vi "mqttServer.vi"() -> ()   [LabVIEW 2019]
uses:
  <vilib>/LabVIEW Open Source Project/MQTT Connection/MQTT_Base/Base Class/MQTT_Base.lvclass/MQTT_Base.ctl
  <vilib>/LabVIEW Open Source Project/MQTT Broker/Server class/Server.lvclass/Server.ctl
  <vilib>/LabVIEW Open Source Project/MQTT Control Packets/Control Packets/PUBLISH/PUBLISH.lvclass
  C:/Program Files (x86)/National Instruments/LabVIEW 2019/vi.lib/LabVIEW Open Source Project/MQTT Control Packets/Control Packets/ControlPacket/ControlPacket.lvclass
  <vilib>/LabVIEW Open Source Project/MQTT Control Packets/Control Packets/ControlPacket/ControlPacket.lvclass/ControlPacket.ctl
  <vilib>/LabVIEW Open Source Project/MQTT TCP Connection/MQTT_TCP/Connection/TCPConnection.lvclass
  C:/Program Files (x86)/National Instruments/LabVIEW 2019/vi.lib/LabVIEW Open Source Project/MQTT Connection/MQTT_Connection/Connection/Connection.lvclass
  <vilib>/LabVIEW Open Source Project/MQTT Broker/Server class/Server.lvclass
  C:/Program Files (x86)/National Instruments/LabVIEW 2019/vi.lib/LabVIEW Open Source Project/MQTT Connection/MQTT_Base/Base Class/MQTT_Base.lvclass
  <vilib>/LabVIEW Open Source Project/Epoch Date & Time/epoch.UNIX/Epoch.UNIX.lvclass
  C:/Program Files (x86)/National Instruments/LabVIEW 2019/vi.lib/LabVIEW Open Source Project/Epoch Date & Time/epoch/Epoch.lvclass
  <vilib>/LabVIEW Open Source Project/Epoch Date & Time/Get Epoch Time.vi
  <vilib>/LabVIEW Open Source Project/MQTT Connection/MQTT_Base/Base Class/MQTT_Base.lvclass
  <vilib>/LabVIEW Open Source Project/MQTT Control Packets/Control Packets/ControlPacket/ControlPacket.lvclass
panel:
  in  "Trace Messages":bool
  out "Error Server":errorcluster
  out "NbConnections":u32
  out "Inbound Log":string
  in  "AutoScroll":bool=TRUE
  in  "Clear Log":bool
  # "Native LabVIEW MQTT Broker"
  # "G Open Source Project for LabVIEW\nhttps://github.com/LabVIEW-Open-Source/LV-MQTT-Broker"
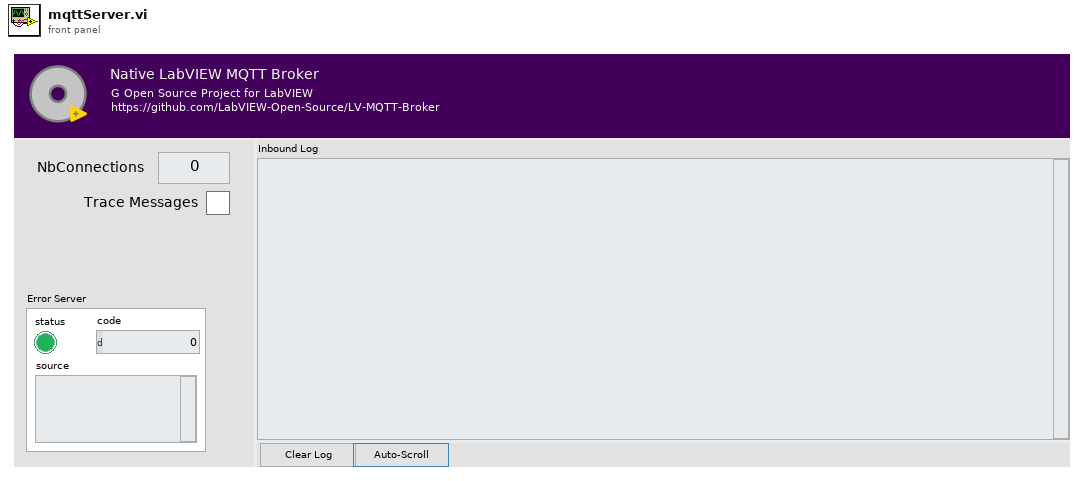
[diagram p1: front panel]
types:
  T1 = typedef "MQTT Base.lvlib/MQTT_Base.lvclass/Public Events -- cluster.ctl" = cluster{"Stop Event":refnum<user-event>, "Error Event":refnum<user-event>, "Inbound Message":refnum<user-event>}
  T2 = typedef "MQTT Server.lvlib/Server.lvclass/Public Events -- cluster.ctl" = cluster{"NbConnections":refnum<user-event>}
  T3 = typedef "MQTT_Control_Packets.lvlib/ControlPacket.lvclass/QualityOfService -- enum.ctl" = enum16{"0 (At Most Once)", "1 (At Least Once)", "2 (Exactly Once)"}
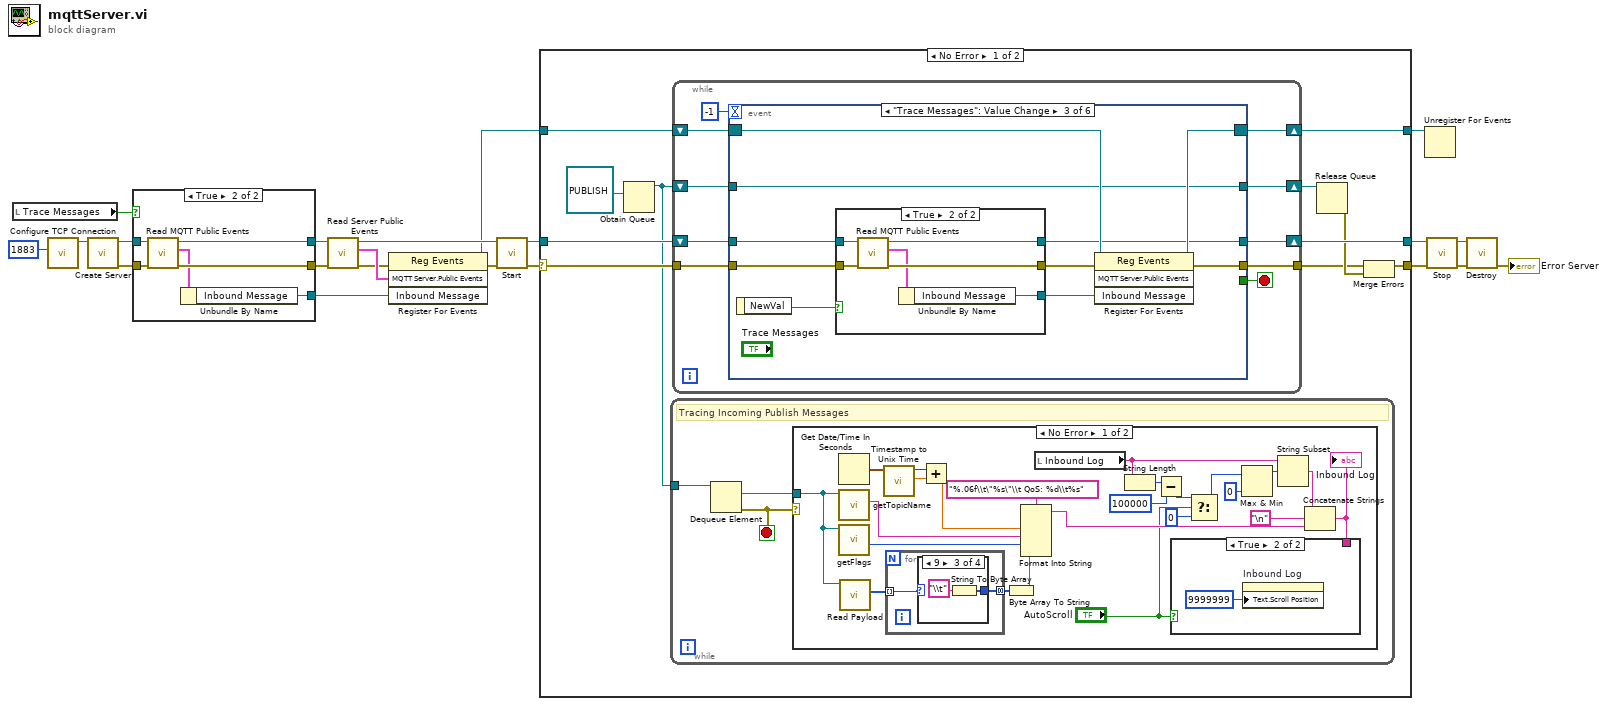
[diagram p0: block diagram]
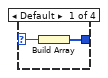
[diagram p4: hidden frame]
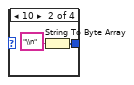
[diagram p5: hidden frame]
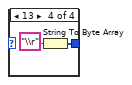
[diagram p6: hidden frame]
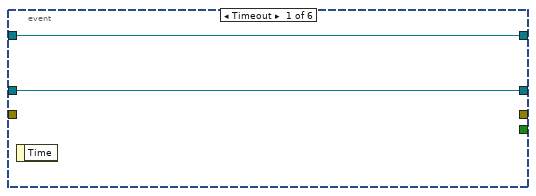
[diagram p8: hidden frame]
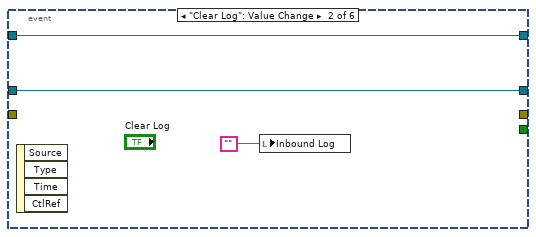
[diagram p9: hidden frame]
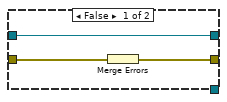
[diagram p10: hidden frame]
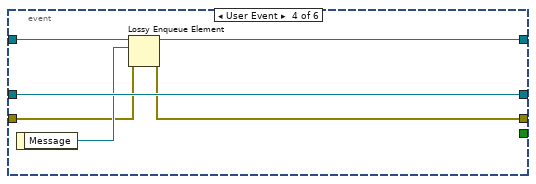
[diagram p11: hidden frame]
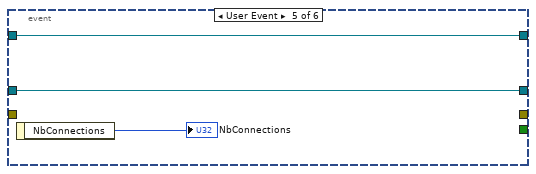
[diagram p12: hidden frame]
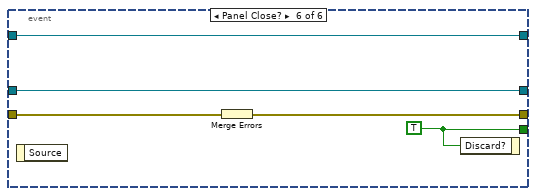
[diagram p13: hidden frame]
diagram:
  n1 = local read "Trace Messages"() -> (w1:bool)
  n2 = call <vilib>:"Configure TCP Connection.vi"("remote port (80)"=u16 1883) -> ("TCPConnection"=w7:refnum<class "TCPConnection.lvclass">)  [unwired: 9 in, 1 out]
  n3 = call <vilib>:"Create Server.vi"("Connection Configuration"=w7) -> ("error out"=w6:errorcluster, "Server"=w4:refnum<class "Server.lvclass">)  [unwired: 9 in]
  n4 = case shown="True" w1 {
    tunnel: w6 -> [w22 w29]
    tunnel: [w22 w28] -> w5
    tunnel: w4 -> [w23 w27]
    tunnel: [w23 w26] -> w3
    tunnel: [_ w24] -> w2
    frame False {
    }
    frame True {
      n5 = call <vilib>:"Read MQTT Public Events.vi"("error in (no error)"=w29, "MQTT_Base in"=w27) -> ("error out"=w28:errorcluster, "MQTT Public Events"=w25:T1, "MQTT_Base out"=w26:refnum<class "Server.lvclass">)  [unwired: 7 in]
      n6 = Unbundle By Name(w25) -> ("Inbound Message"=w24:refnum<user-event>)
    }
  }
  n7 = call <vilib>:"Read Server Public Events.vi"("error in (no error)"=w5, "Server in"=w3) -> ("error out"=w9:errorcluster, "MQTT Server.Public Events"=w10:T2, "Server out"=w13:refnum<class "Server.lvclass">)  [unwired: 7 in]
  n8 = register-events(error in=w9, w10, w2) -> (reference out=w11:refnum<event-registration>, error out=w15:errorcluster)  [unwired: 1 in]
  n9 = call <vilib>:"Start.vi"("error in (no error)"=w15, "MQTT_Base in"=w13) -> ("error out"=w16:errorcluster, "MQTT_Base out"=w14:refnum<class "Server.lvclass">)  [unwired: 7 in, 1 out]
  n10 = case shown="No Error" w16 {
    selector: w16 -> [w36 w127]
    tunnel: w14 -> [w40 w129]
    tunnel: [w39 w129] -> w19
    tunnel: w11 -> [w38 w128]
    tunnel: [w37 w128] -> w12
    tunnel: [w32 w127] -> w21
    frame No Error {
      n11 = Obtain Queue(element data type=refnum<class "PUBLISH.lvclass"> refnum ("Message")) -> (queue out=w31:refnum<queue>)  [unwired: 4 in, 2 out]
      n12 = while {
        tunnel: w31 -> [w43]
        stop <- w42 stop-if-true
        # "Tracing Incoming Publish Messages"
        n13 = Dequeue Element(queue=w43) -> (element=w41:refnum<class "PUBLISH.lvclass">, error out=w42:errorcluster)  [unwired: 2 in, 2 out]
        n14 = case shown="No Error" w42 {
          tunnel: w41 -> [w65 _]
          frame No Error {
            n15 = Get Date/Time In Seconds() -> (seconds since 1Jan1904=w61:timestamp)
            n16 = call <vilib>:"getTopicName.vi"("PUBLISH in"=w65) -> ("Topic"=w67:string)  [unwired: 8 in, 2 out]
            n17 = call-dynamic "getFlags.vi"("PUBLISH in"=w65) -> ("QoS"=w66:T3)  [unwired: 7 in, 3 out]
            n18 = call <vilib>:"Read Payload.vi"("ControlPacket in"=w65) -> ("Payload"=w59:u8[])  [unwired: 9 in, 1 out]
            n19 = call <vilib>:"Timestamp to Unix Time.vi"("Timestamp (now)"=w61) -> ("Fractional Second"=w62:dbl, "Unix Time (s)"=w63:i64)  [unwired: 9 in]
            n20 = for {
              tunnel: w59 -> [w70] mode=indexing
              tunnel: [w69] -> w58 mode=concatenating
              n21 = case shown="9" w70 {
                selector: w70 -> [w72 _ _ _]
                tunnel: [w71 w74 w76 w78] -> w69
                frame Default {
                  n22 = Build Array(w72) -> (w71:u8[])
                }
                frame 10 {
                  n23 = String To Byte Array(string="\\n") -> (unsigned byte array=w74:u8[])
                }
                frame 9 {
                  n24 = String To Byte Array(string="\\t") -> (unsigned byte array=w76:u8[])
                }
                frame 13 {
                  n25 = String To Byte Array(string="\\r") -> (unsigned byte array=w78:u8[])
                }
              }
            }
            n26 = Add(x=w63, y=w62) -> (x+y=w60:dbl)
            n27 = Byte Array To String(unsigned byte array=w58) -> (string=w64:string)
            n28 = Format Into String(format string="%.06f\\t\"%s\"\\t QoS: %d\\t%s", w60, w67, w66, w64) -> (resulting string=w56:string)  [unwired: 2 in, 1 out]
            n29 = local read "Inbound Log"() -> (w53:string)
            n30 = String Length(string=w53) -> (length=w52:i32)
            n31 = Subtract(x=w52, y=100000 ("length (rest)")) -> (x-y=w47:i32)
            n32 = Select(t=w47, s="AutoScroll", f=0 ("y")) -> (s? t:f=w46:i32)
            n33 = Max & Min(x=w46, y=0) -> (max(x,y)=w50:i32)  [unwired: 1 out]
            n34 = String Subset(string=w53, offset (0)=w50) -> (substring=w49:string)  [unwired: 1 in]
            n35 = Concatenate Strings(w49, "\n", w56) -> (w55:string)
            "Inbound Log" <- w55
            n36 = case shown="True" "AutoScroll" {
              tunnel: w55 -> [_ _]
              frame False {
              }
              frame True {
                n37 = property on="Inbound Log" class="Str"("Text.Scroll Position"=u32 9999999) -> ()  [unwired: 2 in, 2 out]
              }
            }
          }
          frame Error {
          }
        }
      }
      n38 = while {
        shift-right: [w85] -> w39
        shift-left: w40 -> [w87]
        tunnel: [w82] -> w33
        tunnel: w36 -> [w81]
        shift-right: [w83] -> w37
        shift-left: w38 -> [w84]
        shift-right: [w79] -> w35
        shift-left: w31 -> [w80]
        stop <- w86 stop-if-true
        n39 = event shown="[2] \"Trace Messages\": Value Change" {
          selector: w84 -> [_ _ w103 _ _ _]
          dyn-events: [_ _ w102 _ _ _] -> w83
          timeout: -1 -> [_ _ _ _ _ _]
          tunnel: w87 -> [w90 w93 w99 w118 w121 w126]
          tunnel: [_ _ _ _ _ w125] -> w86
          tunnel: [w90 w93 w100 w118 w121 w126] -> w85
          tunnel: [_ _ w101 _ _ w123] -> w82
          tunnel: w81 -> [_ _ w97 w113 _ w124]
          tunnel: [_ _ _ w114 _ _] -> _
          tunnel: w80 -> [w89 w92 w94 w117 w119 w122]
          tunnel: [w89 w92 w94 w115 w119 w122] -> w79
          event Timeout {
            n40 = event-data() -> ()  [unwired: 1 in, 1 out]
          }
          event "Clear Log": Value Change {
            n41 = event-data() -> ()  [unwired: 1 in, 4 out]
            n42 = local write "Inbound Log"("") -> ()
          }
          event "Trace Messages": Value Change {
            n43 = event-data() -> ("NewVal"=w95:bool)  [unwired: 1 in]
            n44 = case shown="True" w95 {
              tunnel: [w106 w112] -> w100
              tunnel: w99 -> [w106 w111]
              tunnel: [w105 w110] -> w98
              tunnel: w97 -> [w104 w109]
              tunnel: [_ w108] -> w96
              frame False {
                n45 = Merge Errors(w104) -> (w105:errorcluster)
              }
              frame True {
                n46 = call <vilib>:"Read MQTT Public Events.vi"("error in (no error)"=w109, "MQTT_Base in"=w111) -> ("error out"=w110:errorcluster, "MQTT Public Events"=w107:T1, "MQTT_Base out"=w112:refnum<class "Server.lvclass">)  [unwired: 7 in]
                n47 = Unbundle By Name(w107) -> ("Inbound Message"=w108:refnum<user-event>)
              }
            }
            n48 = register-events(reference=w103, error in=w98, w96) -> (reference out=w102:refnum<event-registration>, error out=w101:errorcluster)  [unwired: 1 in]
          }
          event User Event {
            n49 = event-data() -> ("Message"=w116:refnum<class "PUBLISH.lvclass">)  [unwired: 1 in]
            n50 = Lossy Enqueue Element(queue=w117, element=w116, error in (no error)=w113) -> (queue out=w115:refnum<queue>, error out=w114:errorcluster)  [unwired: 2 out]
          }
          event User Event {
            n51 = event-data() -> ("NbConnections"=→"NbConnections":u32)  [unwired: 1 in]
          }
          event Panel Close? {
            w125 = TRUE ("Discard?")
            n52 = event-data() -> ()  [unwired: 1 in, 1 out]
            n53 = Merge Errors(w124) -> (w123:errorcluster)
            n54 = event-data("Discard?"=w125) -> ()  [unwired: 1 in, 1 out]
          }
        }
      }
      n55 = Release Queue(queue=w35) -> (error out=w34:errorcluster)  [unwired: 2 in, 2 out]
      n56 = Merge Errors(w33, w34) -> (w32:errorcluster)
    }
    frame Error {
    }
  }
  n57 = Unregister For Events(event registration refnum=w12) -> ()  [unwired: 1 in, 1 out]
  n58 = call <vilib>:"Stop.vi"("error in (no error)"=w21, "MQTT_Base in"=w19) -> ("error out"=w20:errorcluster, "MQTT_Base out"=w18:refnum<class "Server.lvclass">)  [unwired: 7 in, 1 out]
  n59 = call <vilib>:"Destroy.vi"("error in (no error)"=w20, "MQTT_Base in"=w18) -> ("error out"=→"Error Server":errorcluster)  [unwired: 8 in, 1 out]
